vi "Get Status.vi"(6 "Axis":T1, 8 "error in (no error)":errorcluster, 11 "Instrument.VRM in":refnum<class "Instrument.OxfordVRM.lvclass">) -> (0 "error out":errorcluster, 1 "Status (ALL)":T2, 2 "Status":string[](array[string]), 3 "Instrument.VRM out":refnum<class "Instrument.OxfordVRM.lvclass">)   [LabVIEW 2019, in "Instrument.OxfordVRM.lvclass"]
doc: "Status Bits:\n[0] = Hold?\n[1] = Ramp to Set?\n[2] = Ramp to Zero?\n[3] = Clamp?"
uses:
  Instrument.OxfordVRM.lvclass
  C:/Program Files (x86)/National Instruments/LabVIEW 2019/user.lib/LevyLab/Instrument Framework/SMOs/Instrument/Instrument.lvclass
  Typedefs/VRM Magnet Axis--Enum.ctl
  Typedefs/Instrument.VRM.Commands-enum.ctl
  <userlib>/LevyLab/Instrument Framework/SMOs/Instrument/Instrument.lvclass/Instrument.ctl
  9aad68f4-b45b-40ed-b713-12b558089732.vi
  9aad68f4-b45b-40ed-b713-12b558089732.vi/c8cd0c6f-915c-46e4-9ceb-c885eaf120ea.vi
  9aad68f4-b45b-40ed-b713-12b558089732.vi/c8cd0c6f-915c-46e4-9ceb-c885eaf120ea.vi/0ceab976-3b6d-4c70-a056-c65624438b19.vi
  <userlib>/LevyLab/Instrument Framework/SMOs/Instrument/API/Send and Receive.vi
  9aad68f4-b45b-40ed-b713-12b558089732.vi/c8cd0c6f-915c-46e4-9ceb-c885eaf120ea.vi/da388c74-ffbc-4760-b489-63bbc35dac72.vi
  <userlib>/LevyLab/Instrument Framework/SMOs/Instrument/Private/Get Client Type.vi
  9aad68f4-b45b-40ed-b713-12b558089732.vi/c8cd0c6f-915c-46e4-9ceb-c885eaf120ea.vi/0ceab976-3b6d-4c70-a056-c65624438b19.vi/b1649572-b77a-4cc9-b4b3-0ac5a01f84bc.vi
  9aad68f4-b45b-40ed-b713-12b558089732.vi/c8cd0c6f-915c-46e4-9ceb-c885eaf120ea.vi/0ceab976-3b6d-4c70-a056-c65624438b19.vi/af59dbd6-f74b-49f0-ac5a-ebfcbb27df43.vi
  9aad68f4-b45b-40ed-b713-12b558089732.vi/c8cd0c6f-915c-46e4-9ceb-c885eaf120ea.vi/da388c74-ffbc-4760-b489-63bbc35dac72.vi/621394de-6b30-4a9a-a0ac-fa3d1c0fc0e8.vi
  9aad68f4-b45b-40ed-b713-12b558089732.vi/c8cd0c6f-915c-46e4-9ceb-c885eaf120ea.vi/da388c74-ffbc-4760-b489-63bbc35dac72.vi/4d9a52a3-3fc2-4304-bf6e-4a3467213c4d.vi
  9aad68f4-b45b-40ed-b713-12b558089732.vi/c8cd0c6f-915c-46e4-9ceb-c885eaf120ea.vi/da388c74-ffbc-4760-b489-63bbc35dac72.vi/621394de-6b30-4a9a-a0ac-fa3d1c0fc0e8.vi/cfc968a8-7cdf-4271-b024-a5daf6eeb4bb.vi
  9aad68f4-b45b-40ed-b713-12b558089732.vi/c8cd0c6f-915c-46e4-9ceb-c885eaf120ea.vi/da388c74-ffbc-4760-b489-63bbc35dac72.vi/621394de-6b30-4a9a-a0ac-fa3d1c0fc0e8.vi/c0eefe53-6a9f-4726-b290-c74d120edb6f.vi
  <userlib>/LevyLab/Instrument Framework/SMOs/Instrument/Private/Get RC Connection Status.vi
  <userlib>/LevyLab/Instrument Framework/SMOs/Instrument/API/Enum to String.vi
  <userlib>/LevyLab/Instrument Framework/SMOs/RemoteControl/API/Send and Receive.vi
  <vilib>/Utility/Data Type/Get Type Information.vi
  <vilib>/JDP Science/JSONtext/JSON text to Variant.vi
  <userlib>/LevyLab/Instrument Framework/SMOs/Instrument/API/Instrument.GetPublicEvents.vi
  <vilib>/JDP Science/JSONtext/Variant to JSON Text.vi
  <vilib>/National Instruments/GUID Generator/Guid Generator.vi
  <userlib>/LevyLab/Instrument Framework/SMOs/Instrument/API/Instrument.MessageToProcess.vi
  <userlib>/LevyLab/Instrument Framework/SMOs/Instrument/Private/Instrument.MessageFromProcess.EventStructure.vi
  <vilib>/JDP Science/JSONtext/LVClass Serializer/JSONtext LVClass Serializer.lvclass
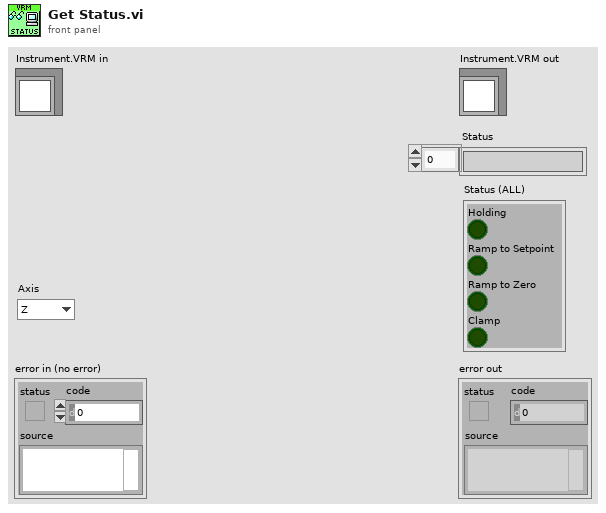
[diagram p1: front panel]
types:
  T1 = typedef "Instrument.OxfordVRM.lvclass/VRM Magnet Axis--Enum.ctl" = enum16{"Z", "X", "Y", "ALL"}
  T2 = cluster{"Holding":bool, "Ramp to Setpoint":bool, "Ramp to Zero":bool, "Clamp":bool}
  T3 = typedef "Instrument.OxfordVRM.lvclass/Instrument.VRM.Commands-enum.ctl" = enum16{"setAction", "setTarget", "setMagnetField", "getStatus", "getTarget", "getMagnetField"}
  T4 = cluster{"[0]":bool, "[1]":bool, "[2]":bool, "[3]":bool}
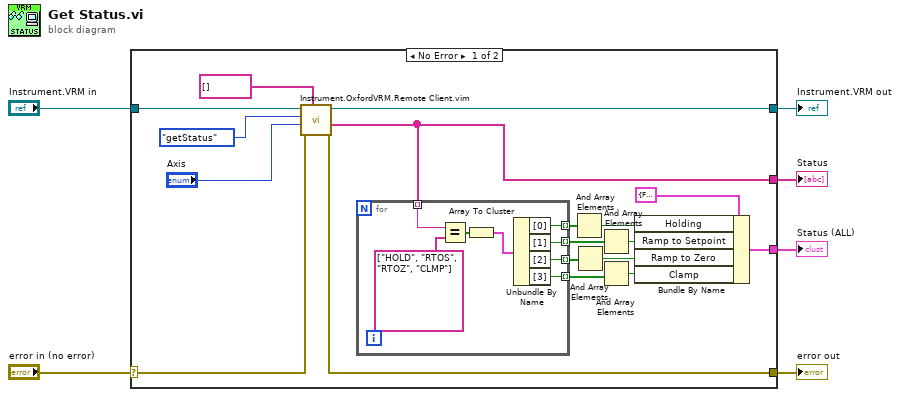
[diagram p0: block diagram]
diagram:
  n1 = case shown="No Error" "error in (no error)" {
    selector: "error in (no error)" -> [w23 w34]
    tunnel: [w7 w34] -> w5
    tunnel: [w21 w33] -> w3
    tunnel: "Instrument.VRM in" -> [w22 w33]
    tunnel: [w19 _] -> w2
    tunnel: [w9 _] -> w1
    frame No Error {
      n2 = call "Instrument.OxfordVRM.Remote Client.vim"("Data Out type"=string[] [], "error in (no error)"=w23, "Data"="Axis", "Commands"=Instrument.VRM.Commands-enum."getStatus", "Instrument.VRM in"=w22) -> ("error out"=w7:errorcluster, "Data out"=w19:string[], "Instrument.VRM out"=w21:refnum<class "Instrument.OxfordVRM.lvclass">)  [unwired: 4 in]
      n3 = for {
        tunnel: w19 -> [w30] mode=indexing
        tunnel: [w28] -> w18 mode=indexing
        tunnel: [w27] -> w17 mode=indexing
        tunnel: [w26] -> w16 mode=indexing
        tunnel: [w25] -> w15 mode=indexing
        n4 = Equal?(x=w30, y=string[] ["HOLD", "RTOS", "RTOZ", "CLMP"] ("Array")) -> (x = y?=w32:bool[])
        n5 = Array To Cluster(array=w32) -> (cluster=w29:T4)
        n6 = Unbundle By Name(w29) -> ("[0]"=w28:bool, "[1]"=w27:bool, "[2]"=w26:bool, "[3]"=w25:bool)
      }
      n7 = And Array Elements(Boolean array=w18) -> (logical AND=w10:bool)
      n8 = And Array Elements(Boolean array=w16) -> (logical AND=w12:bool)
      n9 = And Array Elements(Boolean array=w17) -> (logical AND=w11:bool)
      n10 = And Array Elements(Boolean array=w15) -> (logical AND=w13:bool)
      n11 = Bundle By Name(cluster=T2 {"Holding"=FALSE, "Ramp to Setpoint"=FALSE, "Ramp to Zero"=FALSE, "Clamp"=FALSE} ("Status"), "Holding"=w10, "Ramp to Setpoint"=w11, "Ramp to Zero"=w12, "Clamp"=w13) -> (w9:T2)
    }
    frame Error {
    }
  }
  "error out" <- w5
  "Instrument.VRM out" <- w3
  "Status" <- w2
  "Status (ALL)" <- w1
